vi "SET STOP.vi"(4 "error in (no error)":errorcluster) -> (1 "error out":errorcluster)   [LabVIEW 2012, in "GlobalStop(dev).lvlib"]
uses:
  GlobalStop(dev).lvlib
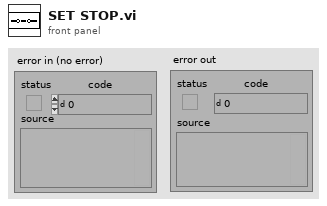
[diagram p1: front panel]
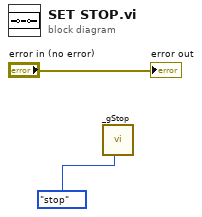
[diagram p0: block diagram]
diagram:
  n1 = call "_gStop.vi"("op"=enum16{"reset", "get", "stop"}."stop") -> ()  [unwired: 10 in, 1 out]
  "error out" <- "error in (no error)"
